vi "Acquire_MultipleData_and_Save_to_File ver 2016.vi"() -> ()   [LabVIEW 2016]
doc: "I. Description:\nThis example demonstrates how to acquire a continuous amount of data (Waveform) using the DAQ device's internal clock.\n\nII. Instructions for Running:\n1. Create an analog input voltage channel.\n2. Set the rate for the sample clock. Additionally, define the sample mode to be continuous.\n3. Call the Start VI to start the acquisition.\n4. Read the waveform data in a loop until the user hits the stop button or an error occurs.\nNote: This example reads data from one or more channels and returns an array of data. Use the Index Array function to access an individual channel of data.\n5. Call the Clear Task VI to clear the Task.\n6. Use the popup dialog box to display an error if any.\n\nIV. I/O Connections Overview:\nMake sure your signal input terminal matches the Physical Channel I/O Control. For further connection information, refer to your hardware reference manual."
uses:
  <vilib>/DAQmx/create/channels.llb/DAQmx Create Channel (AI-Voltage-Basic).vi
  <vilib>/Utility/error.llb/DialogType.ctl
  <vilib>/Utility/file.llb/Write Delimited Spreadsheet (string).vi
  <vilib>/DAQmx/configure/timing.llb/DAQmx Timing (Sample Clock).vi
  <vilib>/DAQmx/read.llb/DAQmx Read (Analog 1D Wfm NChan NSamp).vi
panel:
  out "?":string
  out "Waveform Graph 4":waveform(dbl)(graph)
  out "Waveform Graph 3":waveform(dbl)(graph)
  out "Waveform Graph 2":waveform(dbl)(graph)
  out "Waveform Graph 1":waveform(dbl)(graph)
  in  "Maximum Value 4":dbl=10.0 caption="Maximum Value" format="%0.2f"
  in  "Minimum Value 4":dbl=-10.0 caption="Minimum Value" format="%0.2f"
  in  "Physical Channel 4":tag="Dev2/ai3"
  in  "Maximum Value 3":dbl=10.0 caption="Maximum Value" format="%0.2f"
  in  "Minimum Value 3":dbl=-10.0 caption="Minimum Value" format="%0.2f"
  in  "Physical Channel 3":tag="Dev2/ai2"
  in  "Maximum Value 2":dbl=10.0 caption="Maximum Value" format="%0.2f"
  in  "Minimum Value 2":dbl=-10.0 caption="Minimum Value" format="%0.2f"
  in  "Physical Channel 2":tag="Dev2/ai1"
  out "data":waveform(dbl)[](graph)
  in  "file path (use dialog)":path=path "C:/Users/ankitg/Desktop/test.xls"
  in  "Samples to Read":i32=100
  in  "Physical Channel":tag="Dev2/ai0"
  in  "Minimum Value":dbl=-10.0 format="%0.2f"
  in  "Maximum Value":dbl=10.0 format="%0.2f"
  in  "stop":bool
  in  "Sample Rate":dbl=1000.0 caption="Sample Rate (Hz)" format="%0.2f"
  # "Channel Parameters"
  # "Channel Parameters"
  # "Timing Parameters"
  # "Timing Parameters"
  # "Channel Parameters"
  # "Channel Parameters"
  # "Timing Parameters"
  # "Timing Parameters"
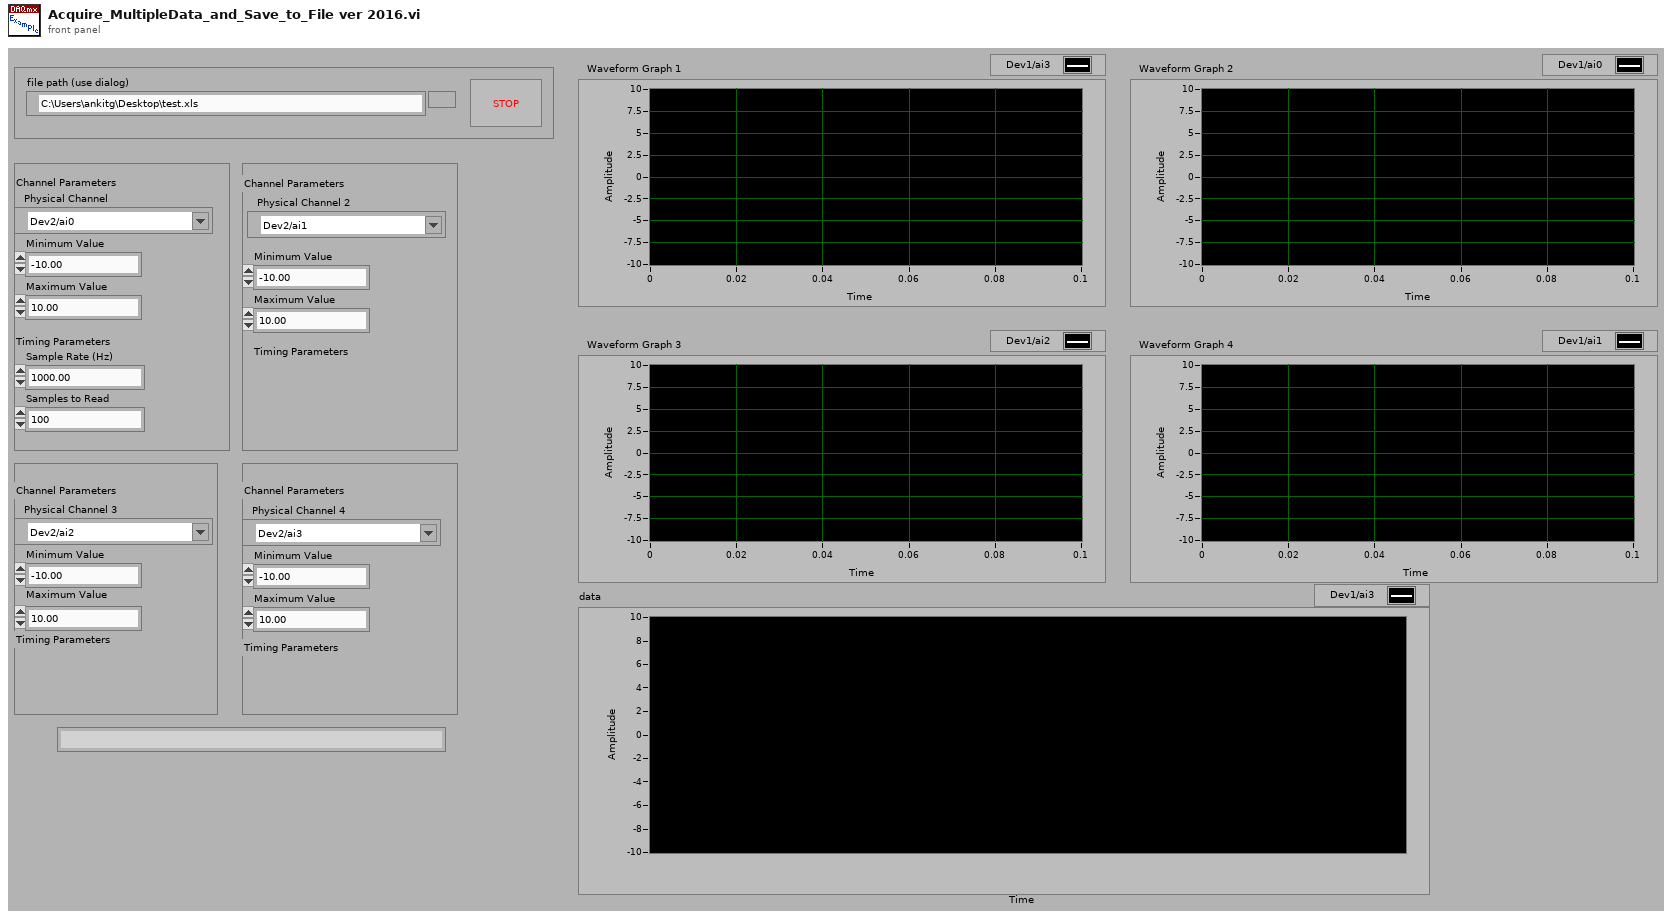
[diagram p1: front panel]
types:
  T1 = typedef "DialogType.ctl" = u16
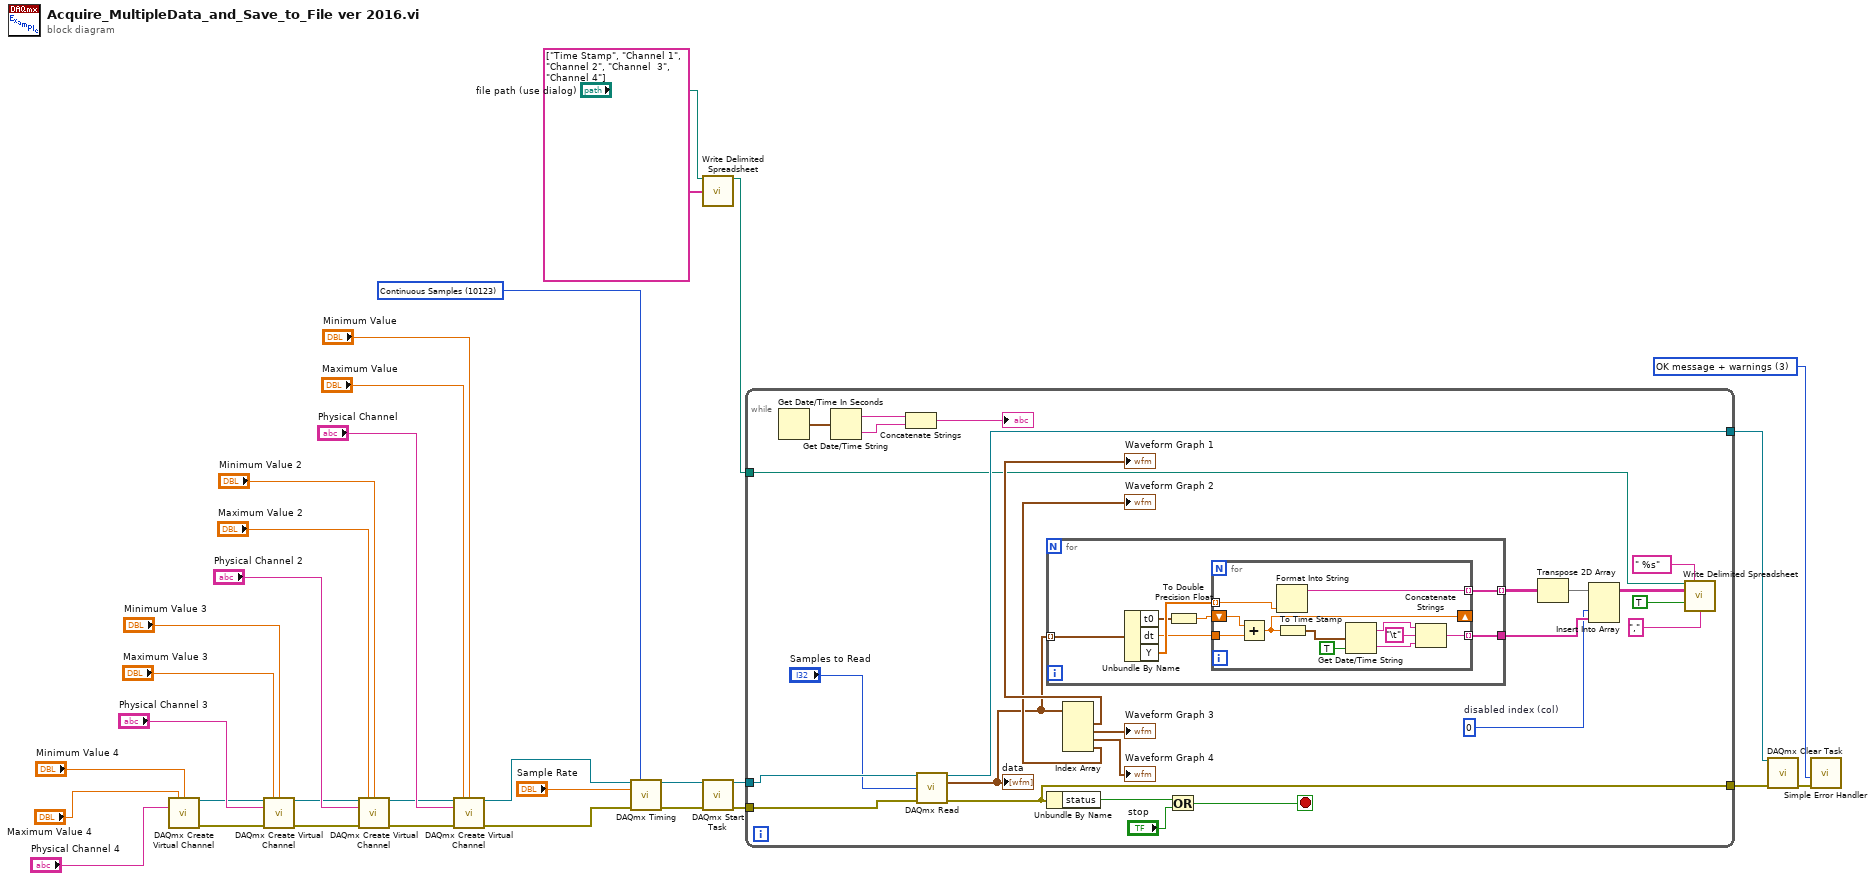
[diagram p0: block diagram]
diagram:
  w23 = T1 3 items=["no dialog", "OK message", "continue or stop message", "OK message + warnings", "continue/stop + warnings"] ("type of dialog (OK msg:1)")
  w8 = 10123 items=["Finite Samples"=10178, "Continuous Samples"=10123] ("sample mode")
  n1 = call-poly <vilib>:"DAQmx Create Virtual Channel.vi"("maximum value"="Maximum Value 4", "minimum value"="Minimum Value 4", "physical channels"="Physical Channel 4") -> ("task out"=w11:refnum<k21>, "error out"=w5:errorcluster)  [unwired: 11 in]
  n2 = call-poly <vilib>:"DAQmx Create Virtual Channel.vi"("task in"=w11, "maximum value"="Maximum Value 3", "minimum value"="Minimum Value 3", "physical channels"="Physical Channel 3", "error in"=w5) -> ("task out"=w10:refnum<k21>, "error out"=w6:errorcluster)  [unwired: 9 in]
  n3 = call-poly <vilib>:"DAQmx Create Virtual Channel.vi"("task in"=w10, "maximum value"="Maximum Value 2", "minimum value"="Minimum Value 2", "physical channels"="Physical Channel 2", "error in"=w6) -> ("task out"=w9:refnum<k21>, "error out"=w7:errorcluster)  [unwired: 9 in]
  n4 = call-poly <vilib>:"DAQmx Create Virtual Channel.vi"("task in"=w9, "maximum value"="Maximum Value", "minimum value"="Minimum Value", "physical channels"="Physical Channel", "error in"=w7) -> ("task out"=w1:refnum<k21>, "error out"=w31:errorcluster)  [unwired: 9 in]
  n5 = call-poly <vilib>:"DAQmx Timing.vi"("task/channels in"=w1, "sample mode"=w8, "rate"="Sample Rate", "error in"=w31) -> ("task out"=w26:refnum<k21>, "error out"=w25:errorcluster)  [unwired: 10 in]
  n6 = call-poly <vilib>:"Write Delimited Spreadsheet.vi"("file path (dialog if empty)"="file path (use dialog)", "1D data"=string[] ["Time Stamp", "Channel 1", "Channel 2", "Channel  3", "Channel 4"]) -> ("new file path (Not A Path if cancelled)"=w2:path)  [unwired: 12 in, 1 out]
  n7 = call <vilib>:"DAQmx Start Task.vi"("task/channels in"=w26, "error in"=w25) -> ("task out"=w29:refnum<k21>, "error out"=w30:errorcluster)  [unwired: 12 in]
  n8 = while {
    tunnel: w30 -> [w59]
    tunnel: w29 -> [w58]
    tunnel: [w57] -> w28
    tunnel: [w53] -> w22
    tunnel: w2 -> [w39]
    stop <- w56 stop-if-true
    w34 = 0  # disabled index (col)
    n9 = Get Date/Time In Seconds() -> (seconds since 1Jan1904=w47:timestamp)
    n10 = Get Date/Time String(seconds (now)=w47) -> (date string=w48:string, time string=w46:string)  [unwired: 2 in]
    n11 = Concatenate Strings(w48, w46) -> (→"?":string)
    n12 = call-poly <vilib>:"DAQmx Read.vi"("task/channels in"=w58, "number of samples per channel"="Samples to Read", "error in"=w59) -> ("task out"=w57:refnum<k21>, "data"=w40:waveform(dbl)[], "error out"=w53:errorcluster)  [unwired: 10 in]
    "data" <- w40
    n13 = for {
      tunnel: w40 -> [w66] mode=indexing
      tunnel: [w60] -> w38 mode=indexing
      tunnel: [w61] -> w37
      n14 = Unbundle By Name(w66) -> ("t0"=w62:timestamp, "dt"=w64:dbl, "Y"=w65:dbl[])
      n15 = To Double Precision Float(number=w62) -> (double precision float=w63:dbl)
      n16 = for {
        tunnel: w65 -> [w77] mode=indexing
        tunnel: [w72] -> w60 mode=indexing
        tunnel: w64 -> [w75]
        shift-right: [w73] -> _
        shift-left: w63 -> [w76]
        tunnel: [w70] -> w61 mode=indexing
        n17 = Add(x=w76, y=w75) -> (x+y=w73:dbl)
        n18 = Format Into String(w77) -> (resulting string=w72:string)  [unwired: 3 in, 1 out]
        n19 = To Time Stamp(1:w73) -> (0:w71:timestamp)
        n20 = Get Date/Time String(seconds (now)=w71, want seconds? (F)=TRUE) -> (date string=w74:string, time string=w68:string)  [unwired: 1 in]
        n21 = Concatenate Strings(w74, "\t", w68) -> (w70:string)
      }
    }
    n22 = Unbundle By Name(w53) -> ("status"=w52:bool)
    n23 = Index Array(array=w40) -> (element #1=→"Waveform Graph 1":waveform(dbl), element #2=→"Waveform Graph 3":waveform(dbl), element #3=→"Waveform Graph 4":waveform(dbl), element #4=→"Waveform Graph 2":waveform(dbl))  [unwired: 4 in]
    n24 = Or(x=w52, y="stop") -> (x .or. y?=w56:bool)
    n25 = Transpose 2D Array(2D array=w38) -> (transposed array=w35:string[][])
    n26 = Insert Into Array(array=w35, index (col)=w34, new element=w37) -> (w36:string[][])  [unwired: 1 in]
    n27 = call-poly <vilib>:"Write Delimited Spreadsheet.vi"("file path (dialog if empty)"=w39, "format (%s)"=" %s", "2D data"=w36, "append to file? (new file:F)"=TRUE, "delimiter (\\t)"="," ("delimiter (\\t)")) -> ()  [unwired: 9 in, 2 out]
  }
  n28 = call <vilib>:"DAQmx Clear Task.vi"("task in"=w28, "error in"=w22) -> ("error out"=w21:errorcluster)  [unwired: 13 in]
  n29 = call <vilib>:"Simple Error Handler.vi"("type of dialog (OK msg:1)"=w23, "error in (no error)"=w21) -> ()  [unwired: 3 in, 5 out]
